vi "ex_GetPacketHeader.vi"(0 "chunk in":string, 1 "Enable":bool, 2 "Decimal Separator":string, 5 "delimiter":string, 7 "file refs in":T1, 9 "file_params":T2 {"time preference" items=["Absolute", "Relative"]; "x_columns" items=["None", "One", "Multiple"]}, 11 "error in":errorcluster) -> (4 "pck special blks":string[](array[string]), 6 "file refs out":T1, 8 "channel info out":T5[](array[typedef]) {"Delta X" format="%.2p"; "X0" format="%<%X\n%x>T"; "Timestamp" format="%<%X\n%x>T"}, 10 "chunk remainder":string, 12 "UUT info":T3, 13 "test info":T4, 14 "notes":string, 15 "error out":errorcluster)   [LabVIEW 2020]
uses:
  <vilib>/express/express shared/ExFile.llb/ex_FileReference.ctl
  <vilib>/express/express shared/ExFile.llb/ex_AllChanInfo.ctl
  <vilib>/express/express input/ExFileReadBlock.llb/ex_ReadFileParams.ctl
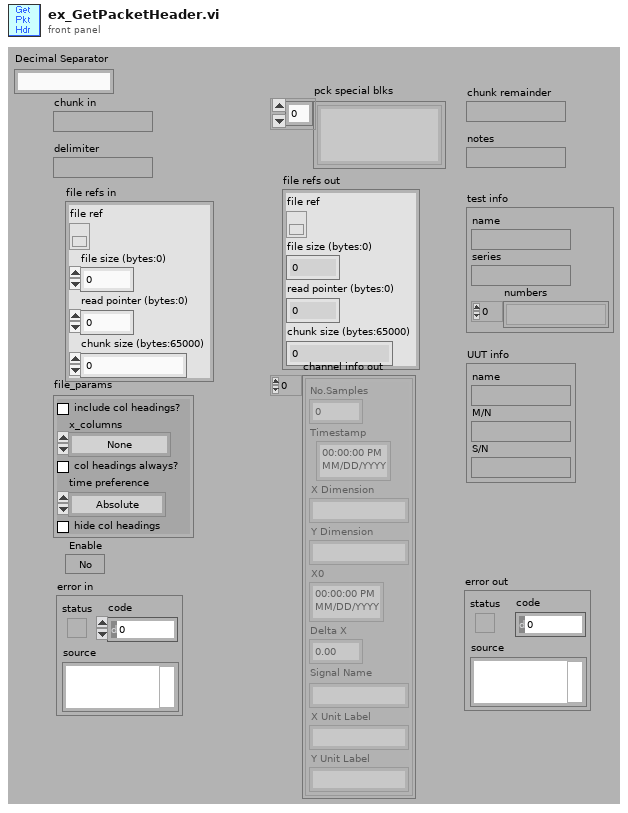
[diagram p1: front panel]
types:
  T1 = typedef "ex_FileReference.ctl" = cluster{"file ref":refnum<file>, "file size (bytes:0)":i32, "read pointer (bytes:0)":i32, "chunk size (bytes:65000)":i32}
  T2 = typedef "ex_ReadFileParams.ctl" = cluster{"include col headings?":bool, "x_columns":u16, "col headings always?":bool, "time preference":u16, "hide col headings":bool}
  T3 = cluster{"name":string, "M/N":string, "S/N":string}
  T4 = cluster{"name":string, "series":string, "numbers":string[]}
  T5 = typedef "ex_AllChanInfo.ctl" = cluster{"No.Samples":i32, "Timestamp":timestamp, "X Dimension":string, "Y Dimension":string, "X0":timestamp, "Delta X":dbl, "Signal Name":string, "X Unit Label":string, "Y Unit Label":string}
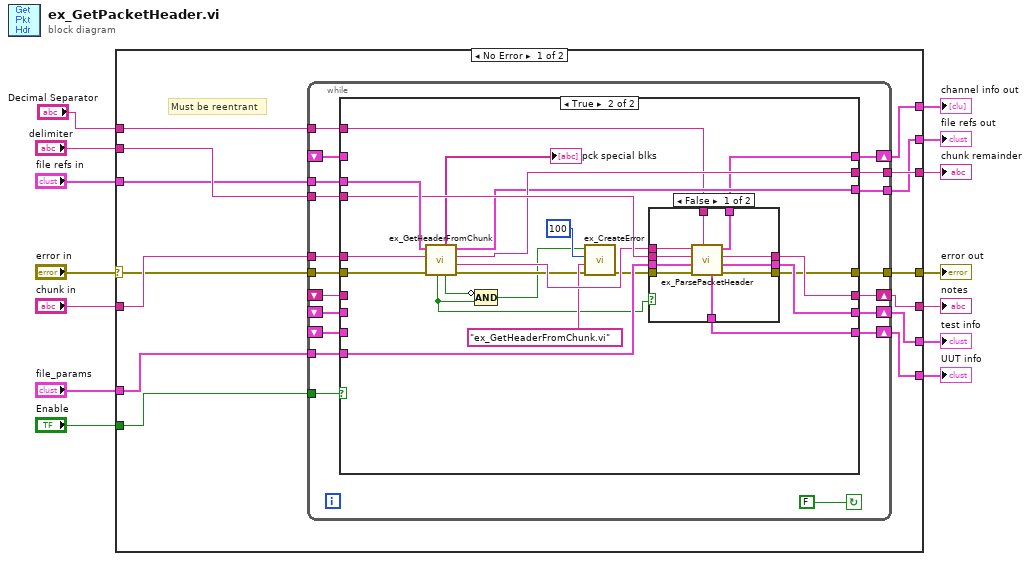
[diagram p0: block diagram]
diagram:
  n1 = case shown="No Error" "error in" {
    selector: "error in" -> [w18 w90]
    tunnel: [w28 w88] -> w14
    tunnel: [w17 _] -> w13
    tunnel: [w27 _] -> w12
    tunnel: [w26 _] -> w11
    tunnel: [w25 _] -> w10
    tunnel: "delimiter" -> [w24 _]
    tunnel: "file refs in" -> [w23 w89]
    tunnel: "chunk in" -> [w22 w88]
    tunnel: "file_params" -> [w21 _]
    tunnel: "Enable" -> [w16 _]
    tunnel: [w20 w90] -> w4
    tunnel: [w19 w89] -> w3
    tunnel: "Decimal Separator" -> [w15 _]
    frame No Error {
      # "Must be reentrant"
      n2 = while {
        tunnel: w22 -> [w47]
        tunnel: w18 -> [w32]
        tunnel: w23 -> [w46]
        tunnel: w24 -> [w45]
        tunnel: w21 -> [w44]
        tunnel: [w39] -> w28
        tunnel: w16 -> [w37]
        shift-right: [w43] -> w25
        shift-left: _ -> [w33]
        shift-right: [w42] -> w26
        shift-left: _ -> [w34]
        shift-right: [w41] -> w27
        shift-left: _ -> [w35]
        shift-right: [w40] -> w17
        shift-left: _ -> [w36]
        tunnel: [w31] -> w20
        tunnel: [w30] -> w19
        tunnel: w15 -> [w29]
        stop <- FALSE continue-if-true
        n3 = case shown="True" w37 {
          tunnel: w47 -> [w48 w76]
          tunnel: w46 -> [w49 w75]
          tunnel: w45 -> [_ w74]
          tunnel: w44 -> [_ w73]
          tunnel: [w51 w72] -> w43
          tunnel: [w52 w71] -> w42
          tunnel: [w53 w70] -> w41
          tunnel: [w54 w59] -> w40
          tunnel: [w48 w69] -> w39
          tunnel: w36 -> [w54 _]
          tunnel: w35 -> [w53 _]
          tunnel: w34 -> [w52 _]
          tunnel: w33 -> [w51 _]
          tunnel: w32 -> [w50 w68]
          tunnel: [w50 w60] -> w31
          tunnel: [w49 w67] -> w30
          tunnel: w29 -> [_ w58]
          frame False {
          }
          frame True {
            n4 = call <vilib>:"ex_GetHeaderFromChunk.vi"("error in (no error)"=w68, "chunk in"=w76, "file ref in"=w75) -> ("error out"=w63:errorcluster, "header"=w66:string, "chunk remainder"=w69:string, "file ref out"=w67:T1, "end of file?"=w57:bool, "special blocks"=→"pck special blks":string[], "no header?"=w55:bool)  [unwired: 2 out]
            n5 = Compound Arithmetic op=AND(invert w57, w55) -> (w56:bool)
            n6 = call <vilib>:"ex_CreateError.vi"("error in (no error)"=w63, "source"="ex_GetHeaderFromChunk.vi", "code"=100, "error?"=w56) -> ("error out"=w62:errorcluster)  [unwired: 7 out]
            n7 = case shown="False" w55 {
              tunnel: w74 -> [w86 _]
              tunnel: w73 -> [w85 _]
              tunnel: [w84 _] -> w72
              tunnel: [w83 _] -> w71
              tunnel: [w82 _] -> w70
              tunnel: w66 -> [w81 _]
              tunnel: w62 -> [w80 w87]
              tunnel: [w79 w87] -> w60
              tunnel: [w78 _] -> w59
              tunnel: w58 -> [w77 _]
              frame False {
                n8 = call <vilib>:"ex_ParsePacketHeader.vi"("Decimal Separator"=w77, "error in (no error)"=w80, "file_params"=w85, "delimiter"=w86, "file header string"=w81) -> ("error out"=w79:errorcluster, "test info"=w83:T4, "notes"=w82:string, "channel info"=w78:T5[], "UUT info"=w84:T3)  [unwired: 2 out]
              }
              frame True {
              }
            }
          }
        }
      }
    }
    frame Error {
    }
  }
  "chunk remainder" <- w14
  "file refs out" <- w3
  "channel info out" <- w13
  "notes" <- w12
  "test info" <- w11
  "UUT info" <- w10
  "error out" <- w4
